vi "RenameClass.vi"(0 "ClassWriterNative.lvclass":refnum<class "ClassWriterNative.lvclass">, 1 "ClassRef":refnum<vi>, 2 "NewClassPath":path, 4 "RelinkWholeProject":bool, 5 "error in (no error)":errorcluster) -> (14 "ClassWriterNative.lvclass":refnum<class "ClassWriterNative.lvclass">, 19 "error out":errorcluster={"status"=TRUE, "code"=1026, "source"="Invoke Node in ClassWriterGOOP300.lvclass:RenameClass.vi"})   [LabVIEW 2016, in "ClassWriterNative.lvclass"]
uses:
  <resource>/Framework/Providers/Open_GDS/ClassProviders/Provider_LvNativeClass/ClassWriterNative_class/ClassWriterNative.lvclass
  <resource>/Framework/Providers/Open_GDS/ClassProviders/Common/ScriptingFunctions/Scripting.lvclass
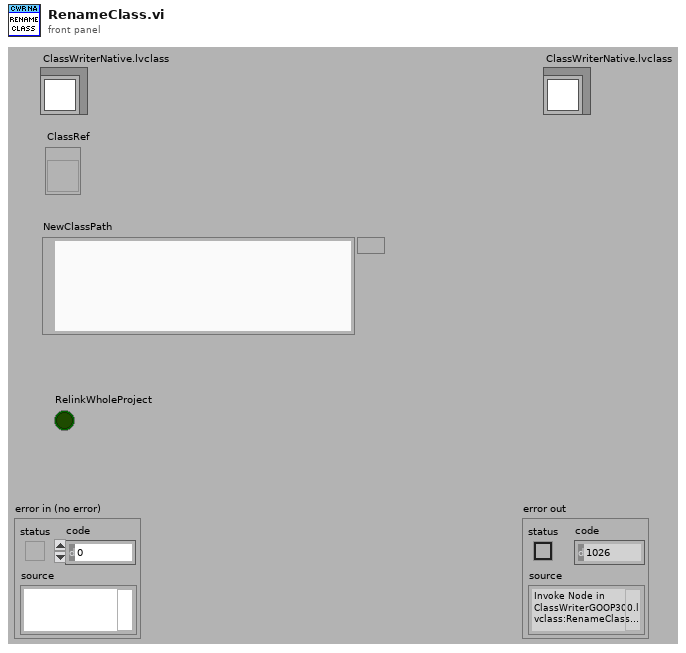
[diagram p1: front panel]
types:
  T1 = cluster{"SubClass":bool, "ClassFiles":path[], "ClassName":string, "ClassFolder":path, "VIs":refnum<vi>[], "TemplateFolder":path, "ViSubDirs":string[], "TemplateName":string, "BaseClassFolder":path, "TemplateClasses":refnum<vi>[], "Application":refnum<vi>}
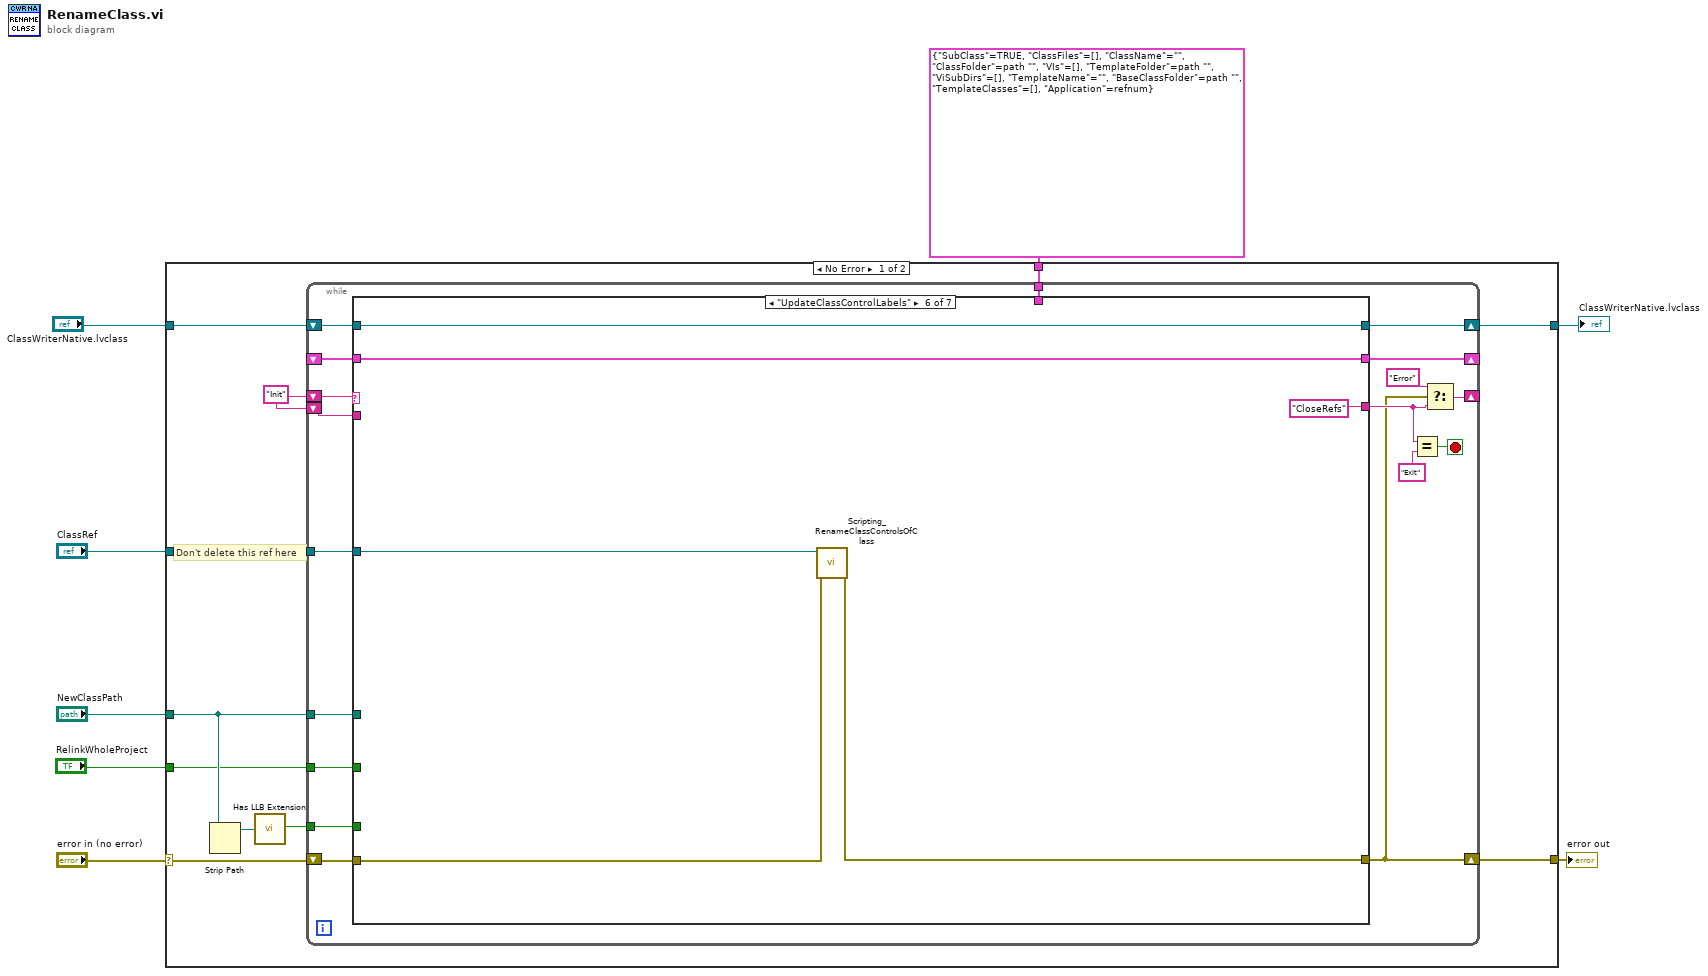
[diagram p0: block diagram]
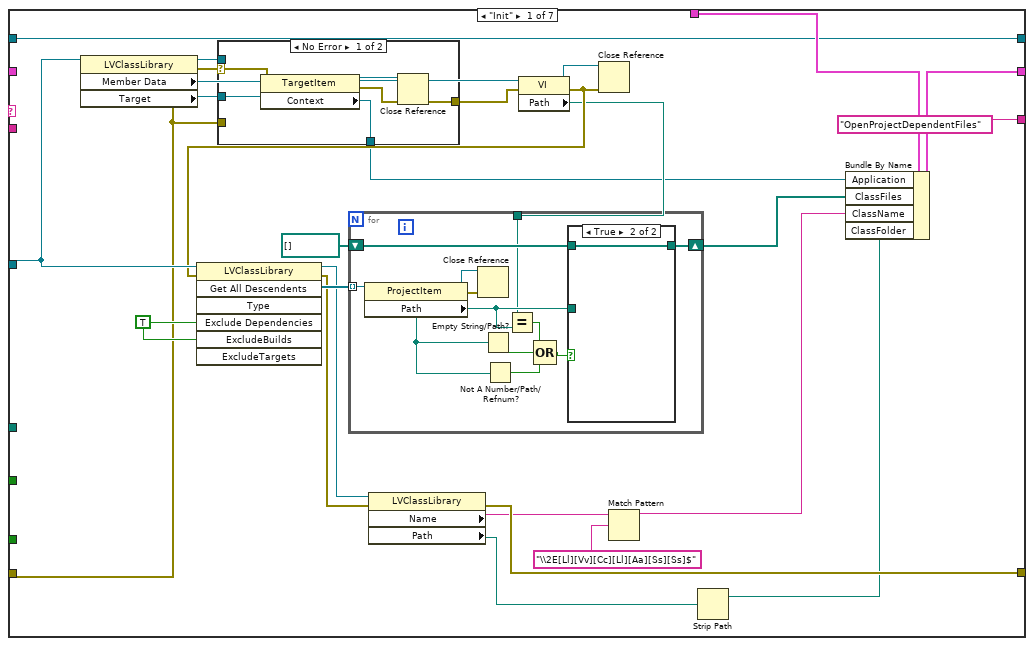
[diagram p2: hidden frame]
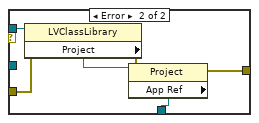
[diagram p3: hidden frame]
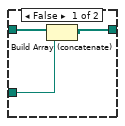
[diagram p4: hidden frame]
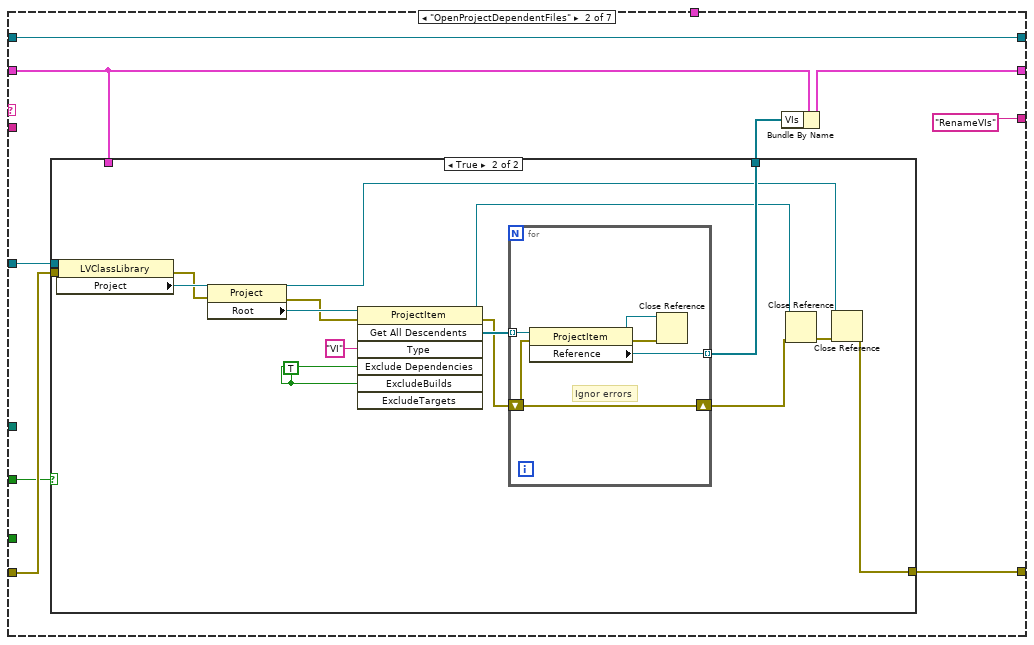
[diagram p5: hidden frame]
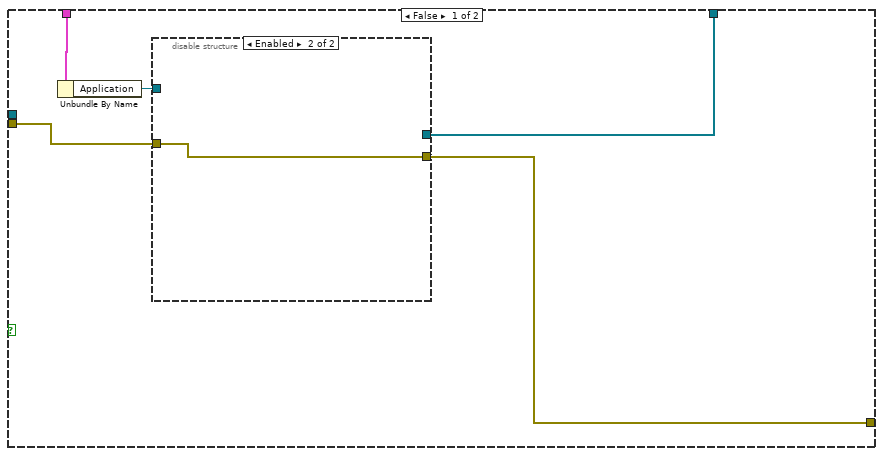
[diagram p6: hidden frame]
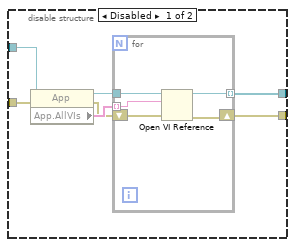
[diagram p7: hidden frame]
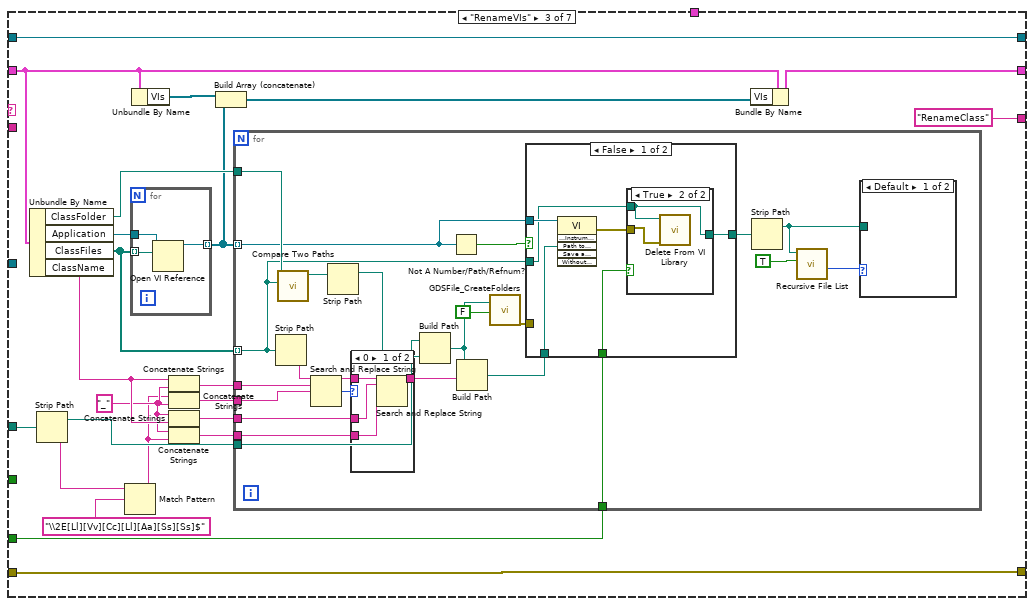
[diagram p8: hidden frame]
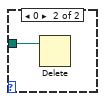
[diagram p10: hidden frame]
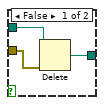
[diagram p11: hidden frame]
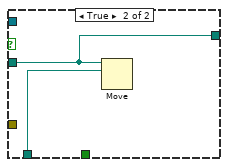
[diagram p12: hidden frame]
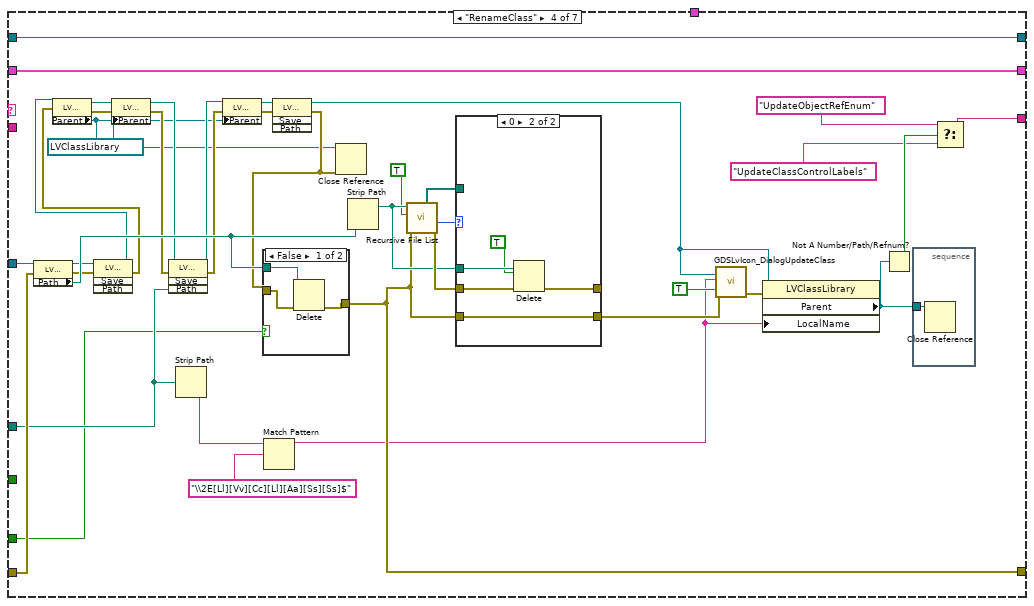
[diagram p13: hidden frame]
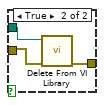
[diagram p14: hidden frame]
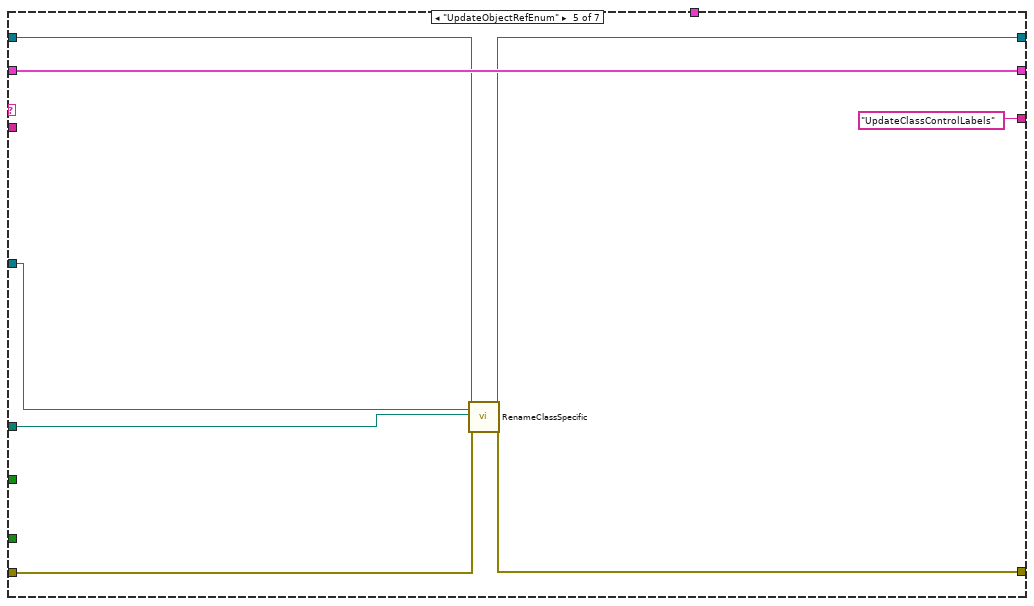
[diagram p16: hidden frame]
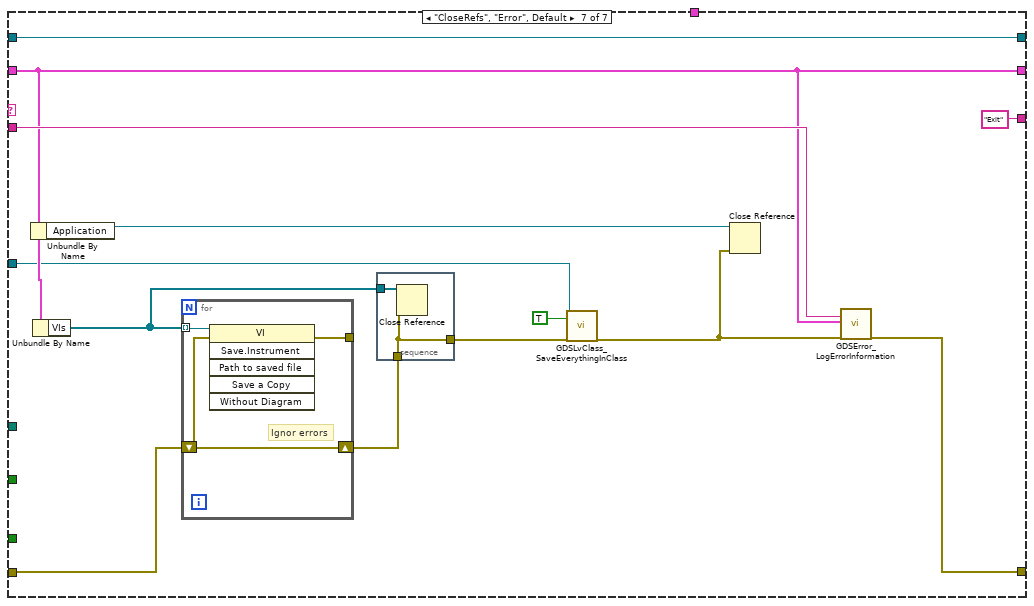
[diagram p17: hidden frame]
diagram:
  n1 = case shown="No Error" "error in (no error)" {
    selector: "error in (no error)" -> [w18 w296]
    tunnel: [w17 w296] -> w8
    tunnel: "ClassRef" -> [w19 _]
    tunnel: T1 {"SubClass"=TRUE, "ClassFiles"=[], "ClassName"="", "ClassFolder"=path "", "VIs"=[], "TemplateFolder"=path "", "ViSubDirs"=[], "TemplateName"="", "BaseClassFolder"=path "", "TemplateClasses"=[], "Application"=refnum} ("output cluster") -> [w16 _]
    tunnel: "NewClassPath" -> [w12 _]
    tunnel: "ClassWriterNative.lvclass" -> [w14 w295]
    tunnel: [w13 w295] -> w2
    tunnel: "RelinkWholeProject" -> [w9 _]
    frame No Error {
      w15 = "Init"
      # "Don't delete this ref here"
      n2 = Strip Path(path=w12) -> (stripped path=w10:path)  [unwired: 1 out]
      n3 = call <vilib>:"Has LLB Extension.vi"("path"=w10) -> ("path to VI library?"=w11:bool)
      n4 = while {
        tunnel: w19 -> [w37]
        shift-right: [w26] -> w17
        shift-left: w18 -> [w36]
        shift-right: [w31] -> _
        shift-left: w15 -> [w27]
        shift-right: [w34] -> _
        shift-left: _ -> [w35]
        tunnel: w16 -> [w29]
        tunnel: w12 -> [w25]
        shift-left: w15 -> [w24]
        shift-right: [w22] -> w13
        shift-left: w14 -> [w23]
        tunnel: w11 -> [w21]
        tunnel: w9 -> [w20]
        stop <- w32 stop-if-true
        n5 = case shown="\"UpdateClassControlLabels\"" w27 {
          tunnel: w35 -> [_ w92 w152 w248 w269 w275 w284]
          tunnel: [w63 w97 w153 w248 w269 w275 w284] -> w34
          tunnel: w37 -> [w50 w99 _ w247 w268 w271 w281]
          tunnel: w36 -> [w38 w98 w161 w246 w266 w273 w288]
          tunnel: [w56 w95 w161 w210 w265 w272 w286] -> w26
          tunnel: ["OpenProjectDependentFiles" "RenameVIs" "RenameClass" w238 "UpdateClassControlLabels" "CloseRefs" "Exit"] -> w28
          tunnel: w29 -> [w62 _ _ _ _ _ _]
          tunnel: w25 -> [_ _ w159 w242 w267 _ _]
          tunnel: w24 -> [_ _ _ _ _ _ w285]
          tunnel: w23 -> [w43 w94 w147 w235 w264 w274 w283]
          tunnel: [w43 w94 w147 w235 w263 w274 w283] -> w22
          tunnel: w21 -> [_ _ w140 w228 _ _ _]
          tunnel: w20 -> [_ w93 _ _ _ _ _]
          frame "Init" {
            w42 = TRUE ("ExcludeDependencies")
            n6 = property class="LVClassLibrary"(reference=w50, error in=w38) -> (reference out=w39:refnum<vi>, error out=w41:errorcluster, "Member Data"=w40:refnum<vi>, "Target"=w46:refnum<vi>)
            n7 = case shown="No Error" w41 {
              selector: w41 -> [w65 _]
              tunnel: w46 -> [w70 _]
              tunnel: [w67 w73] -> w45
              tunnel: [w66 w74] -> w44
              tunnel: w39 -> [_ w76]
              tunnel: w38 -> [_ w71]
              frame No Error {
                n8 = property class="TargetItem"(reference=w70, error in=w65) -> (reference out=w68:refnum<vi>, error out=w69:errorcluster, "Context"=w66:refnum<vi>)
                n9 = Close Reference(reference=w68, error in (no error)=w69) -> (error out=w67:errorcluster)
              }
              frame Error {
                n10 = property class="LVClassLibrary"(reference=w76, error in=w71) -> (error out=w72:errorcluster, "Project"=w75:refnum<vi>)  [unwired: 1 out]
                n11 = property class="Project"(reference=w75, error in=w72) -> (error out=w73:errorcluster, "App Ref"=w74:refnum<vi>)  [unwired: 1 out]
              }
            }
            n12 = property class="VI"(reference=w40, error in=w45) -> (reference out=w48:refnum<vi>, error out=w49:errorcluster, "Path"=w47:path)
            n13 = invoke class="LVClassLibrary" method="Get All Descendents"(reference=w50, error in=w49, "Exclude Dependencies"=w42, "ExcludeBuilds"=w42) -> (reference out=w58:refnum<vi>, error out=w57:errorcluster, "All Descendents"=w61:refnum<vi>[])  [unwired: 3 in, 4 out]
            n14 = for {
              tunnel: w61 -> [w83] mode=indexing
              shift-right: [w86] -> w59
              shift-left: path[] [] -> [w87]
              tunnel: w47 -> [w81]
              n15 = property class="ProjectItem"(reference=w83) -> (reference out=w85:refnum<vi>, error out=w84:errorcluster, "Path"=w82:path)  [unwired: 1 in]
              n16 = Close Reference(reference=w85, error in (no error)=w84) -> ()  [unwired: 1 out]
              n17 = Empty String/Path?(string/path=w82) -> (empty?=w79:bool)
              n18 = Not A Number/Path/Refnum?(number/path/refnum=w82) -> (NaN/Path/Refnum?=w80:bool)
              n19 = Equal?(x=w81, y=w82) -> (x = y?=w78:bool)
              n20 = Compound Arithmetic op=OR(w78, w79, w80) -> (w77:bool)
              n21 = case shown="True" w77 {
                tunnel: w87 -> [w90 w91]
                tunnel: w82 -> [w89 _]
                tunnel: [w88 w91] -> w86
                frame False {
                  n22 = Build Array (concatenate)(w90, w89) -> (w88:path[])
                }
                frame True {
                }
              }
            }
            n23 = property class="LVClassLibrary"(reference=w58, error in=w57) -> (error out=w56:errorcluster, "Name"=w54:string, "Path"=w52:path)  [unwired: 1 out]
            n24 = Close Reference(reference=w48, error in (no error)=w49) -> ()  [unwired: 1 out]
            n25 = Match Pattern(string=w54, regular expression="\\2E[Ll][Vv][Cc][Ll][Aa][Ss][Ss]$" ("string")) -> (before substring=w55:string)  [unwired: 1 in, 3 out]
            n26 = Strip Path(path=w52) -> (stripped path=w51:path)  [unwired: 1 out]
            n27 = Bundle By Name(cluster=w62, "Application"=w44, "ClassFiles"=w59, "ClassName"=w55, "ClassFolder"=w51) -> (w63:T1)
          }
          frame "OpenProjectDependentFiles" {
            n28 = case shown="True" w93 {
              tunnel: w99 -> [_ w134]
              tunnel: w98 -> [w101 w129]
              tunnel: [w105 w126] -> w96
              tunnel: [w104 w120] -> w95
              tunnel: w92 -> [w103 _]
              frame False {
                n29 = Unbundle By Name(w103) -> ("Application"=w102:refnum<vi>)
                n30 = disable-structure shown="Enabled" {
                  disable-tunnel: [w109 _] -> w105
                  disable-tunnel: [w108 w118] -> w104
                  disable-tunnel: w102 -> [w107 _]
                  disable-tunnel: w101 -> [w106 w118]
                  frame Disabled {
                    n31 = property class="App"(reference=w107, error in=w106) -> (reference out=w112:refnum<vi>, error out=w110:errorcluster, "App.AllVIs"=w111:string[])
                    n32 = for {
                      tunnel: w112 -> [w117]
                      tunnel: w111 -> [w116] mode=indexing
                      shift-right: [w114] -> w108
                      shift-left: w110 -> [w115]
                      tunnel: [w113] -> w109 mode=indexing
                      n33 = Open VI Reference(application reference (local)=w117, vi path=w116, error in (no error)=w115) -> (vi reference=w113:refnum<vi>, error out=w114:errorcluster)  [unwired: 3 in]
                    }
                  }
                  frame Enabled {
                  }
                }
              }
              frame True {
                w119 = TRUE ("ExcludeDependencies")
                n34 = property class="LVClassLibrary"(reference=w134, error in=w129) -> (error out=w130:errorcluster, "Project"=w133:refnum<vi>)  [unwired: 1 out]
                n35 = property class="Project"(reference=w133, error in=w130) -> (reference out=w121:refnum<vi>, error out=w128:errorcluster, "Root"=w132:refnum<vi>)
                n36 = invoke class="ProjectItem" method="Get All Descendents"(reference=w132, error in=w128, "Type"="VI", "Exclude Dependencies"=w119, "ExcludeBuilds"=w119) -> (reference out=w123:refnum<vi>, error out=w125:errorcluster, "All Descendents"=w127:refnum<vi>[])  [unwired: 2 in, 4 out]
                n37 = for {
                  tunnel: w127 -> [w139] mode=indexing
                  tunnel: [w138] -> w126 mode=indexing
                  shift-right: [w135] -> w124
                  shift-left: w125 -> [w135]
                  # "Ignor errors"
                  n38 = property class="ProjectItem"(reference=w139, error in=w135) -> (reference out=w136:refnum<vi>, error out=w137:errorcluster, "Reference"=w138:refnum<vi>)
                  n39 = Close Reference(reference=w136, error in (no error)=w137) -> ()  [unwired: 1 out]
                }
                n40 = Close Reference(reference=w123, error in (no error)=w124) -> (error out=w122:errorcluster)
                n41 = Close Reference(reference=w121, error in (no error)=w122) -> (error out=w120:errorcluster)
              }
            }
            n42 = Bundle By Name(cluster=w92, "VIs"=w96) -> (w97:T1)
          }
          frame "RenameVIs" {
            w144 = "_" ("string")
            n43 = Unbundle By Name(w152) -> ("ClassFolder"=w154:path, "Application"=w148:refnum<vi>, "ClassFiles"=w160:path[], "ClassName"=w145:string)
            n44 = Strip Path(path=w159) -> (stripped path=w155:path, name=w158:string)
            n45 = Match Pattern(string=w158, regular expression="\\2E[Ll][Vv][Cc][Ll][Aa][Ss][Ss]$" ("string")) -> (before substring=w143:string)  [unwired: 1 in, 3 out]
            n46 = for {
              tunnel: w160 -> [w208] mode=indexing
              tunnel: [w207] -> w150 mode=indexing
              tunnel: w148 -> [w206]
              n47 = Open VI Reference(application reference (local)=w206, vi path=w208) -> (vi reference=w207:refnum<vi>)  [unwired: 4 in, 1 out]
            }
            n48 = Unbundle By Name(w152) -> ("VIs"=w151:refnum<vi>[])
            n49 = Concatenate Strings(w145, w144) -> (w146:string)
            n50 = Concatenate Strings(w143, w144) -> (w156:string)
            n51 = Concatenate Strings(w144, w145) -> (w142:string)
            n52 = Concatenate Strings(w144, w143) -> (w141:string)
            n53 = Build Array (concatenate)(w151, w150) -> (w149:refnum<vi>[])
            n54 = for {
              tunnel: w150 -> [w172] mode=indexing
              tunnel: w160 -> [w175] mode=indexing
              tunnel: w146 -> [w186]
              tunnel: w156 -> [w185]
              tunnel: w155 -> [w184]
              tunnel: w154 -> [w183]
              tunnel: w142 -> [w169]
              tunnel: w141 -> [w168]
              tunnel: w140 -> [w167]
              n55 = Strip Path(path=w175) -> (name=w182:string)  [unwired: 1 out]
              n56 = call <vilib>:"Compare Two Paths.vi"("Path 2"=w175, "Path 1"=w183) -> ("Relative Path from 1 to 2"=w181:path)  [unwired: 6 in, 3 out]
              n57 = Search and Replace String(input string=w182, search string=w186, replace string=w185) -> (result string=w171:string, number of replacements=w163:i32)  [unwired: 5 in, 2 out]
              n58 = Strip Path(path=w181) -> (stripped path=w180:path)  [unwired: 1 out]
              n59 = case shown="0" w163 {
                tunnel: w171 -> [w190 w191]
                tunnel: [w189 w191] -> w170
                tunnel: w169 -> [w188 _]
                tunnel: w168 -> [w187 _]
                frame 0 {
                  n60 = Search and Replace String(input string=w190, search string=w188, replace string=w187) -> (result string=w189:string)  [unwired: 5 in, 3 out]
                }
                frame Default {
                }
              }
              n61 = Build Path(base path=w184, name or relative path=w180) -> (appended path=w179:path)
              n62 = Not A Number/Path/Refnum?(number/path/refnum=w172) -> (NaN/Path/Refnum?=w177:bool)
              n63 = Build Path(base path=w179, name or relative path=w170) -> (appended path=w174:path)
              n64 = call <resource>:"GDSFile_CreateFolders.vi"("Path"=w179, "Promt if folder\ndoes not exists?"=FALSE ("Promt if folder\ndoes not exists?")) -> ("error out"=w176:errorcluster)  [unwired: 13 in, 4 out]
              n65 = case shown="False" w177 {
                tunnel: w176 -> [_ _]
                tunnel: w175 -> [w194 w204]
                tunnel: w174 -> [w197 w205]
                tunnel: [w196 w204] -> w173
                tunnel: w172 -> [w198 _]
                tunnel: w167 -> [w193 _]
                frame False {
                  n66 = invoke class="VI" method="Save.Instrument"(reference=w198, "Path to saved file"=w197) -> (error out=w195:errorcluster)  [unwired: 4 in, 5 out]
                  n67 = case shown="True" w193 {
                    tunnel: [w201 w203] -> w196
                    tunnel: w195 -> [w200 w202]
                    tunnel: w194 -> [w199 w203]
                    frame False {
                      n68 = Delete(path (use dialog)=w199, error in=w200) -> (deleted path=w201:path)  [unwired: 3 in, 2 out]
                    }
                    frame True {
                      n69 = call <vilib>:"Delete From VI Library.vi"("error in (no error)"=w202, "path"=w203) -> ()  [unwired: 9 in, 1 out]
                    }
                  }
                }
                frame True {
                  n70 = Move(source path=w204, 10:w205) -> ()  [unwired: 3 in, 3 out]
                }
              }
              n71 = Strip Path(path=w173) -> (stripped path=w165:path)  [unwired: 1 out]
              n72 = call <vilib>:"Recursive File List.vi"("Treat LLBs as Folders?"=TRUE, "Folder Path"=w165) -> ("Number of Files"=w164:i32)  [unwired: 5 in, 4 out]
              n73 = case shown="Default" w164 {
                tunnel: w165 -> [_ w192]
                frame Default {
                }
                frame 0 {
                  n74 = Delete(path (use dialog)=w192) -> ()  [unwired: 4 in, 3 out]
                }
              }
            }
            n75 = Bundle By Name(cluster=w152, "VIs"=w149) -> (w153:T1)
          }
          frame "RenameClass" {
            n76 = property class="LVClassLibrary"(reference=w247, error in=w246) -> (reference out=w227:refnum<vi>, error out=w226:errorcluster, "Path"=w229:path)
            n77 = invoke class="LVClassLibrary" method="Save"(reference=w227, error in=w226) -> (reference out=w225:refnum<vi>, error out=w224:errorcluster)  [unwired: 2 in, 2 out]
            n78 = property class="LVClassLibrary"(reference=w225, error in=w224) -> (reference out=w223:refnum<vi>, error out=w222:errorcluster, "Parent"=w212:refnum<vi>)
            n79 = property class="LVClassLibrary"(reference=w223, error in=w222, "Parent"=refnum<vi> refnum ("Parent Class")) -> (reference out=w220:refnum<vi>, error out=w219:errorcluster)
            n80 = invoke class="LVClassLibrary" method="Save"(reference=w220, error in=w219, "Path"=w242) -> (reference out=w218:refnum<vi>, error out=w217:errorcluster)  [unwired: 1 in, 2 out]
            n81 = Strip Path(path=w242) -> (name=w244:string)  [unwired: 1 out]
            n82 = property class="LVClassLibrary"(reference=w218, error in=w217, "Parent"=w212) -> (reference out=w216:refnum<vi>, error out=w215:errorcluster)
            n83 = Match Pattern(string=w244, regular expression="\\2E[Ll][Vv][Cc][Ll][Aa][Ss][Ss]$" ("string")) -> (before substring=w209:string)  [unwired: 1 in, 3 out]
            n84 = invoke class="LVClassLibrary" method="Save"(reference=w216, error in=w215) -> (reference out=w214:refnum<vi>, error out=w213:errorcluster)  [unwired: 2 in, 2 out]
            n85 = case shown="False" w228 {
              tunnel: w213 -> [w251 w253]
              tunnel: w229 -> [w250 w254]
              tunnel: [w249 w252] -> w210
              frame False {
                n86 = Delete(path (use dialog)=w250, error in=w251) -> (error out=w249:errorcluster)  [unwired: 3 in, 2 out]
              }
              frame True {
                n87 = call <vilib>:"Delete From VI Library.vi"("error in (no error)"=w253, "path"=w254) -> ("error out"=w252:errorcluster)  [unwired: 9 in]
              }
            }
            n88 = Close Reference(reference=w212, error in (no error)=w213) -> ()  [unwired: 1 out]
            n89 = Strip Path(path=w229) -> (stripped path=w231:path)  [unwired: 1 out]
            n90 = call <vilib>:"Recursive File List.vi"("error in (no error)"=w210, "Treat LLBs as Folders?"=TRUE, "Folder Path"=w231) -> ("error out"=w233:errorcluster, "Number of Files"=w234:i32, "All Folders"=w232:path[])  [unwired: 4 in, 2 out]
            n91 = case shown="0" w234 {
              tunnel: w231 -> [_ w262]
              tunnel: w233 -> [w257 w259]
              tunnel: [w257 w260] -> _
              tunnel: w232 -> [_ _]
              tunnel: [w256 w258] -> w211
              tunnel: w210 -> [w256 w258]
              frame Default {
              }
              frame 0 {
                n92 = Delete(path (use dialog)=w262, entire hierarchy (F)=TRUE, error in=w259) -> (error out=w260:errorcluster)  [unwired: 2 in, 2 out]
              }
            }
            n93 = call <resource>:"GDSLvIcon_DialogUpdateClass.vi"("ClassPath(FilePath/ProjectTreePath/LvCLassRef)"=w214, "ClassName"=w209, "AutoUpdate"=TRUE, "error in (no error)"=w211) -> ("error out"=w241:errorcluster)  [unwired: 12 in, 3 out]
            n94 = property class="LVClassLibrary"(reference=w214, error in=w241, "LocalName"=w209) -> ("Parent"=w240:refnum<vi>)  [unwired: 2 out]
            n95 = Not A Number/Path/Refnum?(number/path/refnum=w240) -> (NaN/Path/Refnum?=w239:bool)
            n96 = stacked-sequence {
              tunnel: w240 -> [w255]
              frame #0 {
                n97 = Close Reference(reference=w255) -> ()  [unwired: 1 in, 1 out]
              }
            }
            n98 = Select(t="UpdateObjectRefEnum", s=w239, f="UpdateClassControlLabels") -> (s? t:f=w238:string)
          }
          frame "UpdateObjectRefEnum" {
            n99 = call-dynamic "RenameClassSpecific.vi"("ClassWriterNative.lvclass"=w264, "ClassRef"=w268, "NewClassPath"=w267, "error in"=w266) -> ("ClassWriterNative.lvclass"=w263:refnum<class "ClassWriterNative.lvclass">, "error out"=w265:errorcluster)  [unwired: 14 in]
          }
          frame "UpdateClassControlLabels" {
            n100 = call <resource>:"Scripting_RenameClassControlsOfClass.vi"("error in (no error)"=w273, "LVClassLibrary in"=w271) -> ("error out"=w272:errorcluster)  [unwired: 9 in]
          }
          frame "CloseRefs", "Error", Default {
            n101 = Unbundle By Name(w284) -> ("Application"=w287:refnum<vi>)
            n102 = Unbundle By Name(w284) -> ("VIs"=w279:refnum<vi>[])
            n103 = for {
              tunnel: w279 -> [w294] mode=indexing
              shift-right: [w293] -> w278
              shift-left: w288 -> [w293]
              tunnel: [w292] -> _
              # "Ignor errors"
              n104 = invoke class="VI" method="Save.Instrument"(reference=w294, error in=w293) -> (error out=w292:errorcluster)  [unwired: 4 in, 5 out]
            }
            n105 = stacked-sequence {
              tunnel: w279 -> [w291]
              tunnel: w278 -> [w290]
              tunnel: [w290] -> w277
              frame #0 {
                n106 = Close Reference(reference=w291, error in (no error)=w290) -> ()  [unwired: 1 out]
              }
            }
            n107 = call <resource>:"GDSLvClass_SaveEverythingInClass.vi"("ClassRefIn"=w281, "ForceResaving(False)"=TRUE, "error in"=w277) -> ("error out"=w282:errorcluster)  [unwired: 15 in, 1 out]
            n108 = Close Reference(reference=w287, error in (no error)=w282) -> ()  [unwired: 1 out]
            n109 = call <resource>:"GDSError_LogErrorInformation.vi"("State"=w285, "LocalVariableData"=w284, "error in (no error)"=w282) -> ("error out"=w286:errorcluster)  [unwired: 16 in]
          }
        }
        n110 = Equal?(x=w28, y="Exit") -> (x = y?=w32:bool)
        n111 = Select(t="Error", s=w26, f=w28) -> (s? t:f=w31:string)
      }
    }
    frame Error {
    }
  }
  "ClassWriterNative.lvclass" <- w2
  "error out" <- w8
